vi "Source Voltage and Measure using DMM.vi"() -> ()   [LabVIEW 2021]
uses:
  <instrlib>/niDCPower/nidcpower.llb/niDCPower Source Mode.ctl
  <instrlib>/niDCPower/nidcpower.llb/niDCPower Output Function.ctl
  <instrlib>/Agilent 3446X Series/Public/Data/Read (Single Point).vi
  <instrlib>/Agilent 3446X Series/Agilent 3446X Series.lvlib
panel:
  in  "Absolute Resolution (1E-6)":dbl=1e-06
  in  "Agilent DMM":refnum<visa-resource-name>
  in  "Manual Range (1)":dbl=1.0
  out "Measurement using DMM":dbl
  in  "error in":errorcluster
  out "error out":errorcluster
  out "Voltage Measurement":dbl
  out "Current Measurement":dbl
  in  "Current Limit Range":dbl=0.01 format="%.3p"
  in  "Voltage Level Range":dbl=6.0 format="%.5p"
  in  "Current Limit":dbl=0.01 format="%.3p"
  in  "Voltage Level":dbl=2.0 format="%.5p"
  in  "Vin SMU Channel":string="0"
  in  "Vin SMU":refnum<k15>="Dev1"
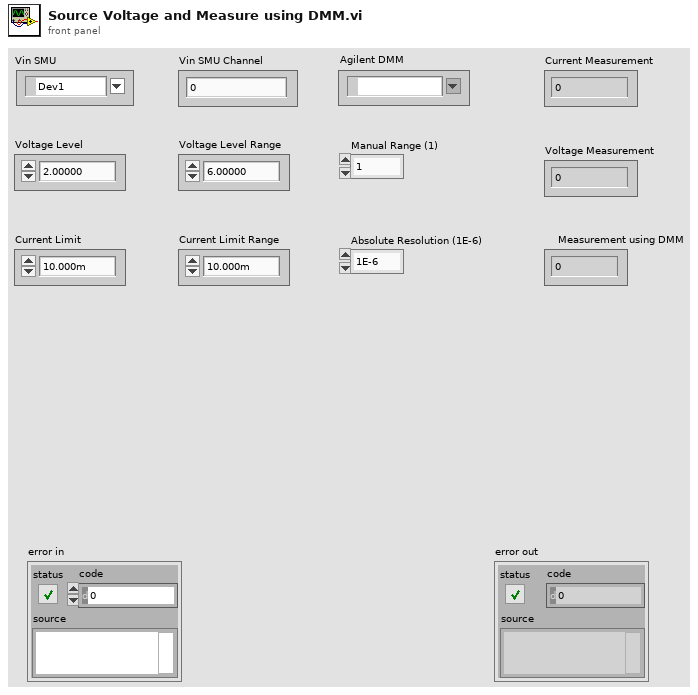
[diagram p1: front panel]
types:
  T1 = typedef "niDCPower Output Function.ctl" = i32
  T2 = typedef "niDCPower Source Mode.ctl" = i32
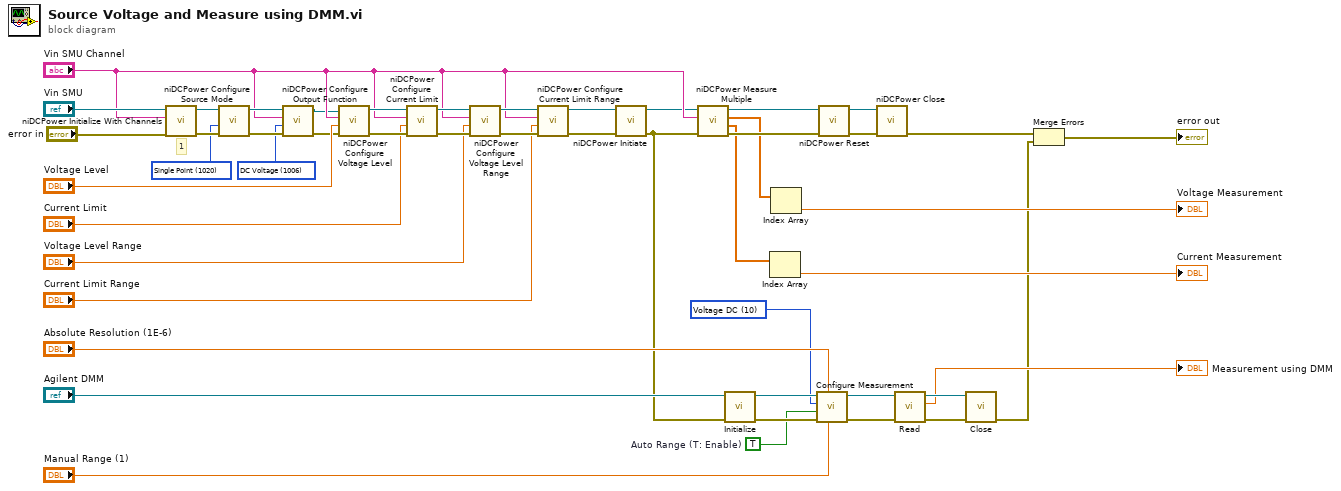
[diagram p0: block diagram]
diagram:
  w1 = TRUE  # Auto Range (T: Enable)
  w5 = 10 items=["Continuity", "Current AC", "Current DC", "Diode", "Frequency", "Resistance 4-wire", "Period", "Resistance 2-wire", "Temperature", "Voltage AC", "Voltage DC", "Voltage DC Ratio", "Capacitance"] ("Measurement Function (10: Voltage DC)")
  w22 = T1 1006 items=["DC Voltage"=1006, "DC Current"=1007, "Pulse Voltage"=1049, "Pulse Current"=1050] ("output function")
  w37 = T2 1020 items=["Single Point"=1020, "Sequence"=1021] ("source mode")
  # "1"
  n1 = call <instrlib>:"niDCPower Initialize With Channels.vi"("error in (no error)"="error in", "channels"="Vin SMU Channel", "resource name"="Vin SMU") -> ("error out"=w41:errorcluster, "instrument handle out"=w40:refnum<k15>)  [unwired: 2 in, 5 out]
  n2 = call <instrlib>:"niDCPower Configure Source Mode.vi"("error in (no error)"=w41, "source mode"=w37, "instrument handle"=w40) -> ("error out"=w39:errorcluster, "instrument handle out"=w38:refnum<k15>)  [unwired: 7 out]
  n3 = call <instrlib>:"niDCPower Configure Output Function.vi"("error in (no error)"=w39, "output function"=w22, "channel name"="Vin SMU Channel", "instrument handle"=w38) -> ("error out"=w23:errorcluster, "instrument handle out"=w24:refnum<k15>)  [unwired: 6 out]
  n4 = call <instrlib>:"niDCPower Configure Voltage Level.vi"("error in (no error)"=w23, "voltage level"="Voltage Level", "channel name"="Vin SMU Channel", "instrument handle"=w24) -> ("error out"=w46:errorcluster, "instrument handle out"=w47:refnum<k15>)  [unwired: 6 out]
  n5 = call <instrlib>:"niDCPower Configure Current Limit.vi"("error in (no error)"=w46, "current limit"="Current Limit", "channel name"="Vin SMU Channel", "instrument handle"=w47) -> ("error out"=w36:errorcluster, "instrument handle out"=w35:refnum<k15>)  [unwired: 1 in, 5 out]
  n6 = call <instrlib>:"niDCPower Configure Voltage Level Range.vi"("error in (no error)"=w36, "voltage level range"="Voltage Level Range", "channel name"="Vin SMU Channel", "instrument handle"=w35) -> ("error out"=w34:errorcluster, "instrument handle out"=w33:refnum<k15>)  [unwired: 6 out]
  n7 = call <instrlib>:"niDCPower Configure Current Limit Range.vi"("error in (no error)"=w34, "current limit range"="Current Limit Range", "channel name"="Vin SMU Channel", "instrument handle"=w33) -> ("error out"=w27:errorcluster, "instrument handle out"=w28:refnum<k15>)  [unwired: 6 out]
  n8 = call <instrlib>:"niDCPower Initiate.vi"("error in (no error)"=w27, "instrument handle"=w28) -> ("error out"=w4:errorcluster, "instrument handle out"=w25:refnum<k15>)  [unwired: 2 in, 6 out]
  n9 = call <instrlib>:"niDCPower Measure Multiple.vi"("error in (no error)"=w4, "channel name"="Vin SMU Channel", "instrument handle"=w25) -> ("error out"=w29:errorcluster, "current measurements"=w19:dbl[], "voltage measurements"=w17:dbl[], "instrument handle out"=w30:refnum<k15>)  [unwired: 5 out]
  n10 = call <instrlib>:"Initialize.vi"("error in (no error)"=w4, "VISA resource name"="Agilent DMM") -> ("error out"=w14:errorcluster, "VISA resource name out"=w15:refnum<visa-resource-name>)  [unwired: 3 in, 5 out]
  n11 = Index Array(array=w19) -> (element=→"Current Measurement":dbl)  [unwired: 1 in]
  n12 = Index Array(array=w17) -> (element=→"Voltage Measurement":dbl)  [unwired: 1 in]
  n13 = call <instrlib>:"Configure Measurement.vi"("Manual Range (1)"="Manual Range (1)", "Absolute Resolution (1E-6)"="Absolute Resolution (1E-6)", "error in (no error)"=w14, "Auto Range (T: Enable)"=w1, "Measurement Function (10: Voltage DC)"=w5, "VISA resource name"=w15) -> ("error out"=w10:errorcluster, "VISA resource name out"=w11:refnum<visa-resource-name>)  [unwired: 4 out]
  n14 = call <instrlib>:"niDCPower Reset.vi"("error in (no error)"=w29, "instrument handle"=w30) -> ("error out"=w43:errorcluster, "instrument handle out"=w44:refnum<k15>)  [unwired: 2 in, 6 out]
  n15 = call <instrlib>:"niDCPower Close.vi"("error in (no error)"=w43, "instrument handle"=w44) -> ("error out"=w20:errorcluster)  [unwired: 9 out]
  n16 = call-poly <instrlib>:"Read.vi"("error in (no error)"=w10, "VISA resource name"=w11) -> ("error out"=w13:errorcluster, "Measurement"=→"Measurement using DMM":dbl, "VISA resource name out"=w12:refnum<visa-resource-name>)  [unwired: 7 out]
  n17 = call <instrlib>:"Close.vi"("error in (no error)"=w13, "VISA resource name"=w12) -> ("error out"=w2:errorcluster)  [unwired: 9 out]
  n18 = Merge Errors(w20, w2) -> (→"error out":errorcluster)
